vi "GetParam.vi"(8 "error in (no error)":errorcluster caption="entrée d'erreur (pas d'erreur)", 11 "Cosine_similarity.lvclass":refnum<class "Cosine_similarity.lvclass">) -> (0 "error out":errorcluster caption="sortie d'erreur", 2 "cosine_similarity":cluster{"dense_output":bool}={"dense_output"=TRUE}, 3 "Cosine_similarity.lvclass":refnum<class "Cosine_similarity.lvclass">)   [LabVIEW 2020, in "Cosine_similarity.lvclass"]
doc: "Get Parameters"
uses:
  Cosine_similarity.lvclass
  Cosine_similarity.lvclass/Cosine_similarity.ctl
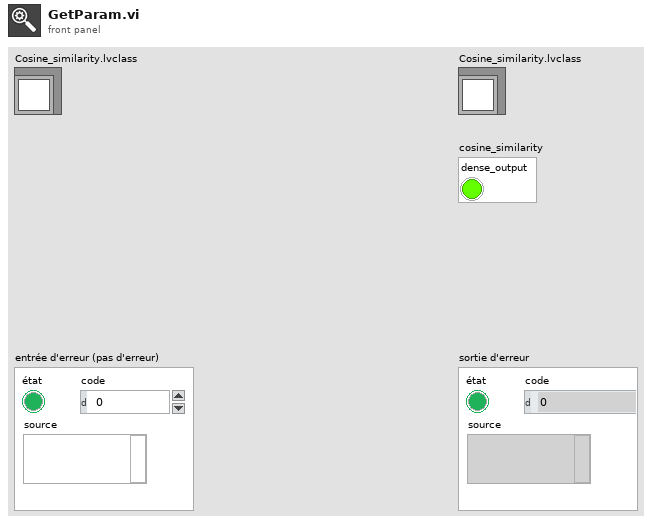
[diagram p1: front panel]
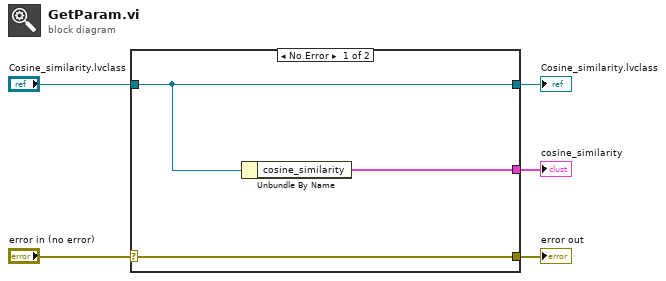
[diagram p0: block diagram]
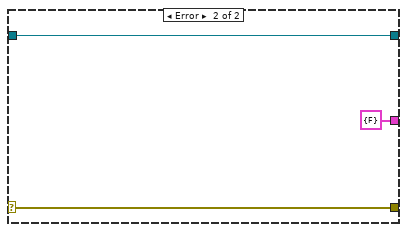
[diagram p2: hidden frame]
diagram:
  n1 = case shown="No Error" "error in (no error)" {
    selector: "error in (no error)" -> [w8 w10]
    tunnel: [w8 w10] -> w4
    tunnel: [w7 w11] -> w2
    tunnel: "Cosine_similarity.lvclass" -> [w7 w11]
    tunnel: [w6 cluster{"dense_output":bool} {"dense_output"=FALSE} ("cosine_similarity")] -> w1
    frame No Error {
      n2 = Unbundle By Name(w7) -> ("cosine_similarity"=w6:cluster{"dense_output":bool})
    }
    frame Error {
    }
  }
  "error out" <- w4
  "Cosine_similarity.lvclass" <- w2
  "cosine_similarity" <- w1
